vi "Untitled 2.vi"() -> ()   [LabVIEW 2015]
panel:
  in  "stop":bool
  out "Numeric":dbl
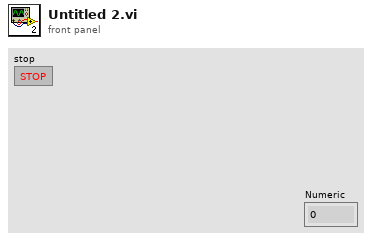
[diagram p1: front panel]
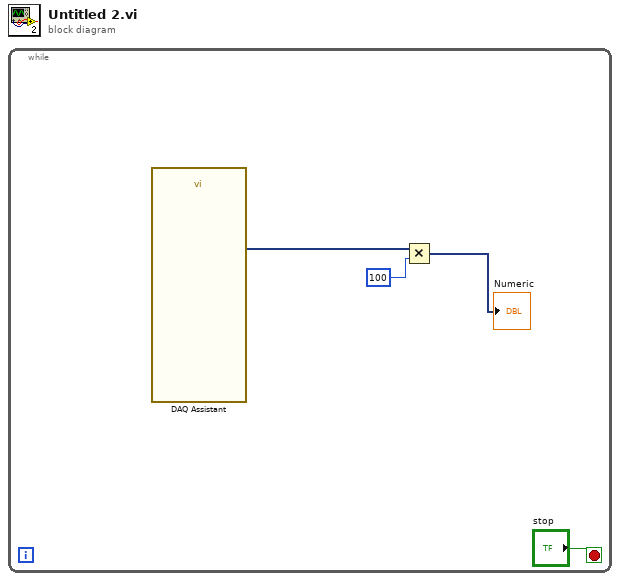
[diagram p0: block diagram]
diagram:
  n1 = while {
    stop <- "stop" stop-if-true
    n2 = call "DAQ Assistant"() -> ("data"=w4:dynamicdata)  [unwired: 17 in, 2 out]
    n3 = Multiply(x=w4, y=100) -> (x*y=→"Numeric":dynamicdata)
  }
